vi "Open.vi"(8 "error in (no error)":errorcluster, 9 "Operation":T1, 10 "Path":path, 11 "Data.PG in":refnum<class "LV-Data.PGSQL.lvclass">) -> (0 "error out":errorcluster, 3 "Data.PG out":refnum<class "LV-Data.PGSQL.lvclass">)   [LabVIEW 2019, in "LV-Data.PGSQL.lvclass"]
uses:
  LV-Data.PGSQL.lvclass
  LV-Data/Typedefs/Operation--enum.ctl
  LV-Data.PGSQL.lvclass/LV-Data.PGSQL.ctl
  LV-Data/LV-Data.lvclass
  <vilib>/JDP Science/PostgreSQL Library/Connection/PQ Connection.lvclass
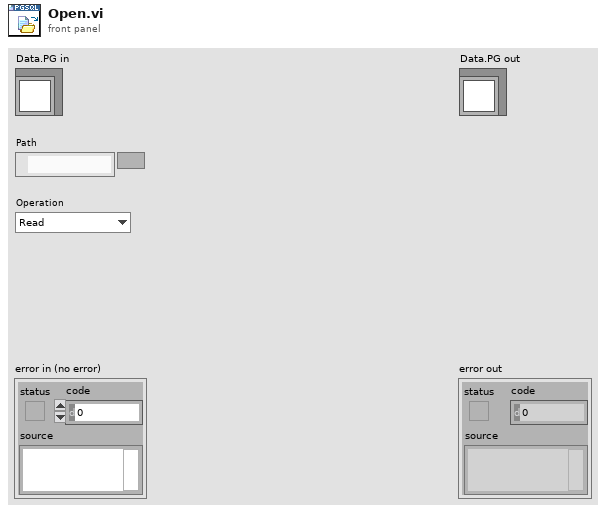
[diagram p1: front panel]
types:
  T1 = typedef "LV-Data.lvclass/Operation--enum.ctl" = enum16{"Read", "Write", "Write + Append"}
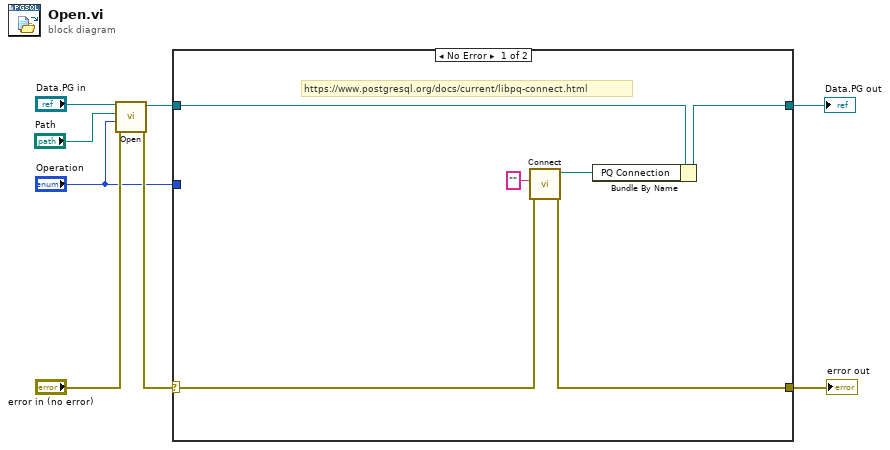
[diagram p0: block diagram]
diagram:
  n1 = call-parent "Open.vi"("error in (no error)"="error in (no error)", "Operation"="Operation", "Path"="Path", "Data in"="Data.PG in") -> ("error out"=w6:errorcluster, "Data out"=w4:refnum<class "LV-Data.PGSQL.lvclass">)  [unwired: 6 in]
  n2 = case shown="No Error" w6 {
    selector: w6 -> [w9 w16]
    tunnel: [w12 w16] -> w5
    tunnel: w4 -> [w11 w15]
    tunnel: [w14 w15] -> w3
    tunnel: "Operation" -> [_ _]
    frame No Error {
      # "https://www.postgresql.org/docs/current/libpq-connect.html"
      n3 = call <vilib>:"Connect.vi"("error in (no error)"=w9, "Connection Strings"="") -> ("error out"=w12:errorcluster, "PQ Connection out"=w13:refnum<class "PQ Connection.lvclass">)  [unwired: 8 in]
      n4 = Bundle By Name(cluster=w11, "PQ Connection"=w13) -> (w14:refnum<class "LV-Data.PGSQL.lvclass">)
    }
    frame Error {
    }
  }
  "error out" <- w5
  "Data.PG out" <- w3
